vi "OP400ZP_Param_ConfZENplusOP100.vi"(8 "errin":errorcluster, 10 "Chaîne":string, 11 "pathin":path) -> (0 "errout":errorcluster, 3 "VISA OUT":cluster{"BT3562":string, "MX5060":string})   [LabVIEW 2020]
uses:
  <vilib>/Utility/config.llb/Read Key (String).vi
  <vilib>/Utility/config.llb/NI_LVConfig.lvlib
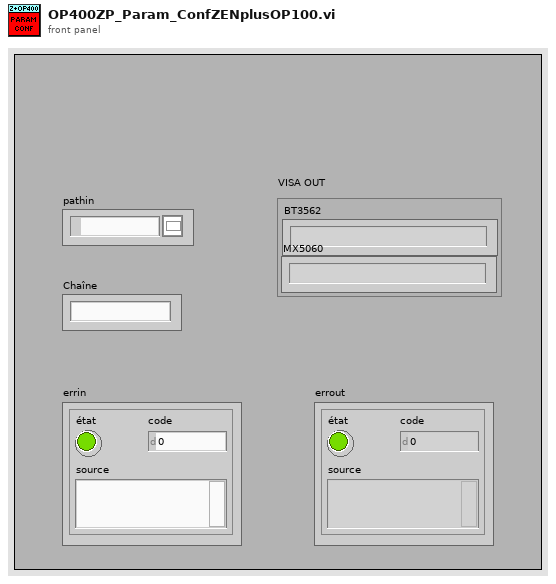
[diagram p1: front panel]
types:
  T1 = typedef "NI_LVConfig.lvlib/Config Data RefNum.ctl" = refnum<k1>
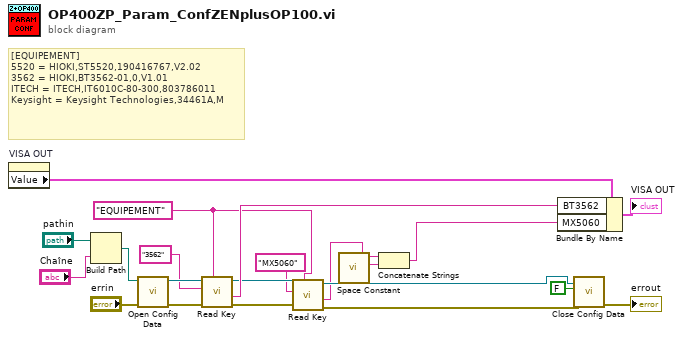
[diagram p0: block diagram]
diagram:
  w4 = "EQUIPEMENT" ("section")
  # "[EQUIPEMENT]\n5520 = HIOKI,ST5520,190416767,V2.02\n3562 = HIOKI,BT3562-01,0,V1.01\nITECH = ITECH,IT6010C-80-300,803786011\nKeysight = Keysight Technologies,34461A,M"
  n1 = property on="VISA OUT" class="Clust (strict)"() -> ("Value"=w10:cluster{"BT3562":string, "MX5060":string})  [unwired: 2 in, 2 out]
  n2 = Build Path(base path="pathin", name or relative path="Chaîne") -> (appended path=w18:path)
  n3 = call <vilib>:"Open Config Data.vi"("error in (no error)"="errin", "configuration file path"=w18) -> ("error out"=w20:errorcluster, "refnum"=w21:T1)  [unwired: 7 in, 1 out]
  n4 = call-poly <vilib>:"Read Key.vi"("section"=w4, "error in (no error)"=w20, "key"="3562", "refnum"=w21) -> ("error out"=w9:errorcluster, "value"=w14:string, "refnum out"=w8:T1)  [unwired: 4 in, 1 out]
  n5 = call-poly <vilib>:"Read Key.vi"("section"=w4, "error in (no error)"=w9, "key"="MX5060", "refnum"=w8) -> ("error out"=w5:errorcluster, "value"=w3:string, "refnum out"=w6:T1)  [unwired: 4 in, 1 out]
  n6 = call <vilib>:"Space Constant.vi"() -> ("String"=w2:string)
  n7 = Concatenate Strings(w3, w2) -> (w1:string)
  n8 = Bundle By Name(cluster=w10, "BT3562"=w14, "MX5060"=w1) -> (→"VISA OUT":cluster{"BT3562":string, "MX5060":string})
  n9 = call <vilib>:"Close Config Data.vi"("error in (no error)"=w5, "write file if changed (T)"=FALSE, "refnum"=w6) -> ("error out"=→"errout":errorcluster)  [unwired: 7 in, 1 out]
